vi "QueryServer_AddTestDataTypesEvent.vi"(11 "gRPCid in":T1) -> (2 "QueryServer_TestDataTypes":refnum<user-event>, 3 "gRPCid":T1)   [LabVIEW 2019, in "labview-grpc-query-server.lvlib"]
uses:
  labview-grpc-query-server.lvlib
  QueryServer_InvokeEventData.ctl
  QueryServer_gRPCid.ctl
  a66ee327-264b-4784-bac1-fff8ba4a2692.vi
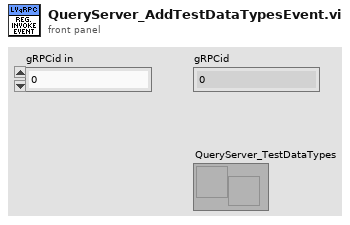
[diagram p1: front panel]
types:
  T1 = typedef "labview-grpc-query-server.lvlib/QueryServer_gRPCid.ctl" = u64
  T2 = typedef "labview-grpc-query-server.lvlib/QueryServer_InvokeEventData.ctl" = cluster{"gRPCid":T1}
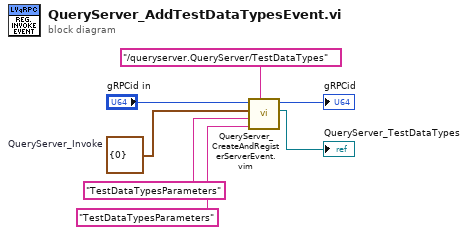
[diagram p0: block diagram]
diagram:
  w4 = T2 {"gRPCid"=0}  # QueryServer_Invoke
  n1 = call "QueryServer_CreateAndRegisterServerEvent.vim"("name"="/queryserver.QueryServer/TestDataTypes", "Response Metadata Name"="TestDataTypesParameters" ("Name"), "Request Metadata Name"="TestDataTypesParameters" ("Name"), "event in"=w4, "gRPCid in"="gRPCid in") -> ("event"=→"QueryServer_TestDataTypes":refnum<user-event>, "gRPCid"=→"gRPCid":T1)  [unwired: 5 in]
